vi "DBL_2_STRING_ARRAY.vi"(1 "Insect-data-array":dbl[][](array[numeric])) -> (0 "Insect-data-array":string[][](array[string]))   [LabVIEW 2024]
doc: "Convertes the double insect-data-array to a sting insect-data-array with headlines"
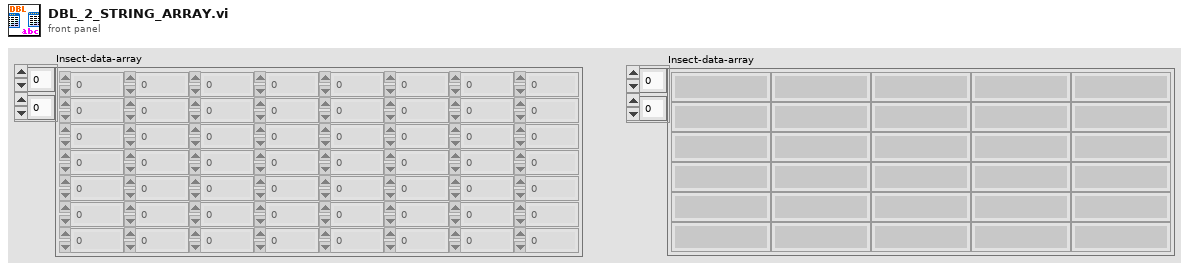
[diagram p1: front panel]
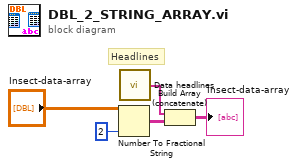
[diagram p0: block diagram]
diagram:
  # "Headlines"
  n1 = Number To Fractional String(number="Insect-data-array", precision (6)=i16 2) -> (F-format string=w3:string[][])  [unwired: 2 in]
  n2 = call "Data headlines.vi"() -> ("Headlines (vertical array)"=w5:string[])
  n3 = Build Array (concatenate)(w5, w3) -> (→"Insect-data-array":string[][])
